vi "CamCalibration (SubVI).vi"(8 "error in":errorcluster, 10 "Image Dst":T1, 11 "Image In":T1) -> (0 "error out":errorcluster, 3 "Image Out":T1)   [LabVIEW 2019]
uses:
  <vilib>/vision/Image Controls.llb/IMAQ Image.ctl
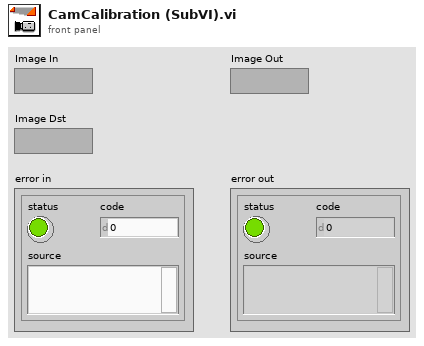
[diagram p1: front panel]
types:
  T1 = typedef "IMAQ Image.ctl" = refnum<image>
  T2 = cluster{"Origin Pixel":cluster{"X":sgl, "Y":sgl}, "X Axis Pixel":cluster{"X":sgl, "Y":sgl}, "Axis Reference":u32}
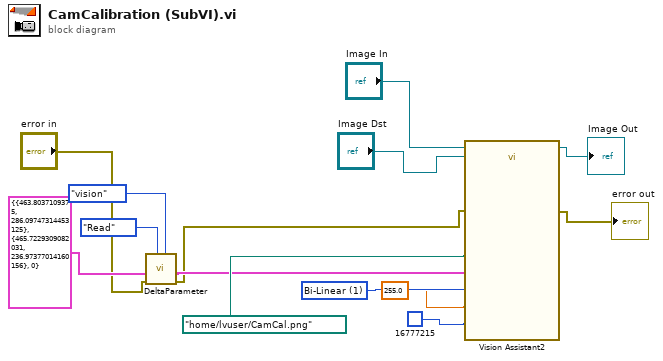
[diagram p0: block diagram]
diagram:
  w7 = u32 1 items=["Zero Order", "Bi-Linear", "Quadratic", "Cubic Spline"] ("Interpolation Type (Image Correction 1)")
  n1 = call "DeltaParameter.vi"("parameter"=enum16{"angle", "robot", "vision"}."vision", "mode"=enum16{"Read", "Write"}."Read", "error in (no error)"="error in", "視覺參數write"=T2 {"Origin Pixel"={"X"=463.8037, "Y"=286.09747}, "X Axis Pixel"={"X"=465.72293, "Y"=236.97377}, "Axis Reference"=0} ("Calibration Axis Info (Image Calibration 1)")) -> ("error out"=w1:errorcluster, "視覺參數read"=w3:T2)  [unwired: 3 in, 3 out]
  n2 = call "Vision Assistant2"("Image In"="Image In", "Image Dst"="Image Dst", "Calibration Axis Info (Image Calibration 1)"=w3, "Interpolation Type (Image Correction 1)"=w7, "Replace Value (Image Correction 1)"=sgl 255.0, "Color Replace Value (Image Correction 1)"=u32 16777215, "File Path (Image Calibration 1)"=path "/home/lvuser/CamCal.png", "error in"=w1) -> ("Image Out"=→"Image Out":T1, "error out"=→"error out":errorcluster)  [unwired: 18 in]
